vi "_get_lambda.vi"(8 "error in (no error)":errorcluster, 11 "UV-VIS_AVANTES in":refnum<class "UV-VIS_AVANTES.lvclass">) -> (0 "error out":errorcluster, 2 "a_pWaveLength":dbl[](array[numeric]), 3 "UV-VIS_AVANTES out":refnum<class "UV-VIS_AVANTES.lvclass">)   [LabVIEW 2020, in "UV-VIS_AVANTES.lvclass"]
uses:
  UV-VIS_AVANTES.lvclass
  C:/Dev/TRANCON/Classes/Detector/Detector.lvclass
  Detector.lvclass/Detector.ctl
  UV-VIS_AVANTES.lvclass/UV-VIS_AVANTES.ctl
  Detector.lvclass
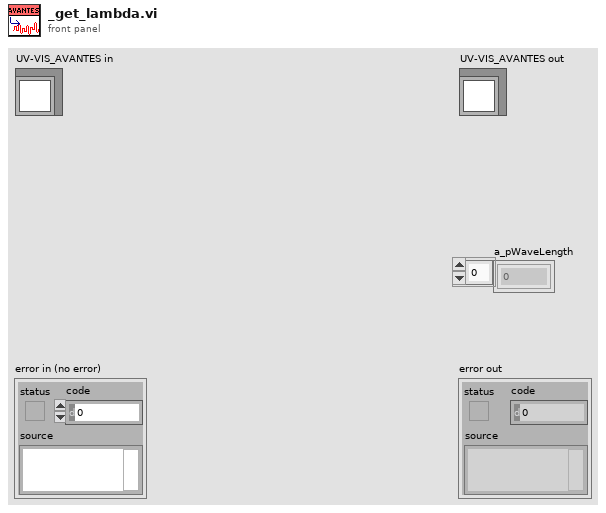
[diagram p1: front panel]
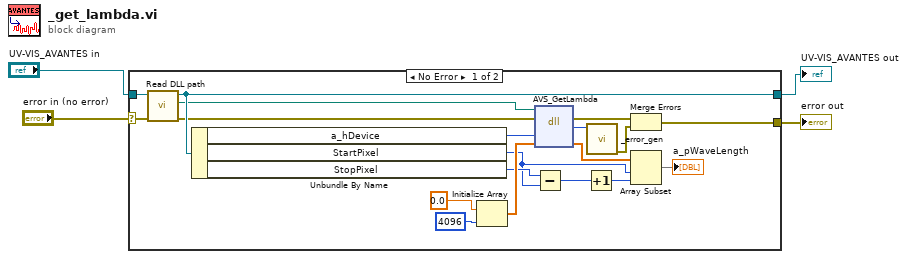
[diagram p0: block diagram]
diagram:
  n1 = case shown="No Error" "error in (no error)" {
    selector: "error in (no error)" -> [w22 w25]
    tunnel: [w7 w25] -> w3
    tunnel: [w21 w24] -> w1
    tunnel: "UV-VIS_AVANTES in" -> [w23 w24]
    frame No Error {
      n2 = call "Read DLL path.vi"("error in (no error)"=w22, "Detector in"=w23) -> ("error out"=w19:errorcluster, "DLL path"=w20:path, "Detector out"=w21:refnum<class "UV-VIS_AVANTES.lvclass">)  [unwired: 7 in]
      n3 = Unbundle By Name(w21) -> ("a_hDevice"=w15:i32, "StartPixel"=w10:u16, "StopPixel"=w11:u16)
      n4 = Initialize Array(0.0, 4096 ("dimension size")) -> (w16:dbl[])
      n5 = dll-call lib="C:/AvaSpecX64-DLL_9.4/examples/LabView/LabViewSingleChan/avaspec.dll" fn="AVS_GetLambda"(path in=w20, error in=w19, "a_hDevice"=w15, "a_pWaveLength"=w16) -> (error out=w6:errorcluster, "return type"=w5:i32, "a_pWaveLength"=w14:dbl[])  [unwired: 2 in, 1 out]
      n6 = Subtract(x=w11, y=w10) -> (x-y=w12:u16)
      n7 = Increment(x=w12) -> (x+1=w9:u16)
      n8 = call "_error_gen.vi"("return type"=w5) -> ("error out"=w8:errorcluster)  [unwired: 10 in]
      n9 = Merge Errors(w6, w8) -> (w7:errorcluster)
      n10 = Array Subset(array=w14, index=w10, length=w9) -> (→"a_pWaveLength":dbl[])
    }
    frame Error {
    }
  }
  "error out" <- w3
  "UV-VIS_AVANTES out" <- w1
